vi "Untitled 1.vi"(11 "ZXing Options in":refnum<class "ZXing Options.lvclass">) -> (3 "ZXing Options out":refnum<class "ZXing Options.lvclass">)   [LabVIEW 2020, in "feature_detection.lvlib" / "ZXing Options.lvclass"]
uses:
  ZXing Options.lvclass
  ZXing Options.lvclass/ZXing Options.ctl
panel:
  in  "Ring":u8(ring) items=["ASCII", "ISO8859_1", "ISO8859_2", "ISO8859_3", "ISO8859_4", "ISO8859_5", "ISO8859_6", "ISO8859_7", "ISO8859_8", "ISO8859_9", "ISO8859_10", "ISO8859_11", "ISO8859_13", "ISO8859_14", "ISO8859_15", "ISO8859_16", "Cp437", "Cp1250", "Cp1251", "Cp1252", "Cp1256", "Shift_JIS", "Big5", "GB2312", "GB18030", "EUC_JP", "EUC_KR", "UTF16BE", "UTF8", "UTF16LE", "UTF32BE", "UTF32LE", "BINARY"]
  out "string array":string[](array[string])
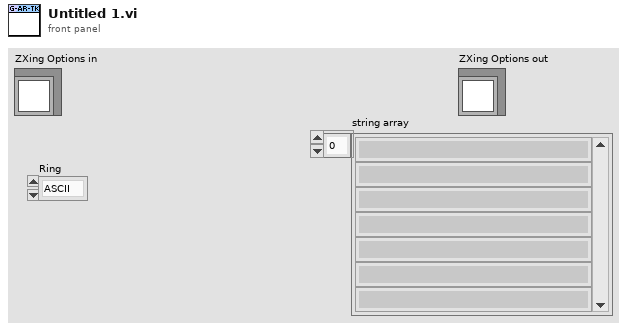
[diagram p1: front panel]
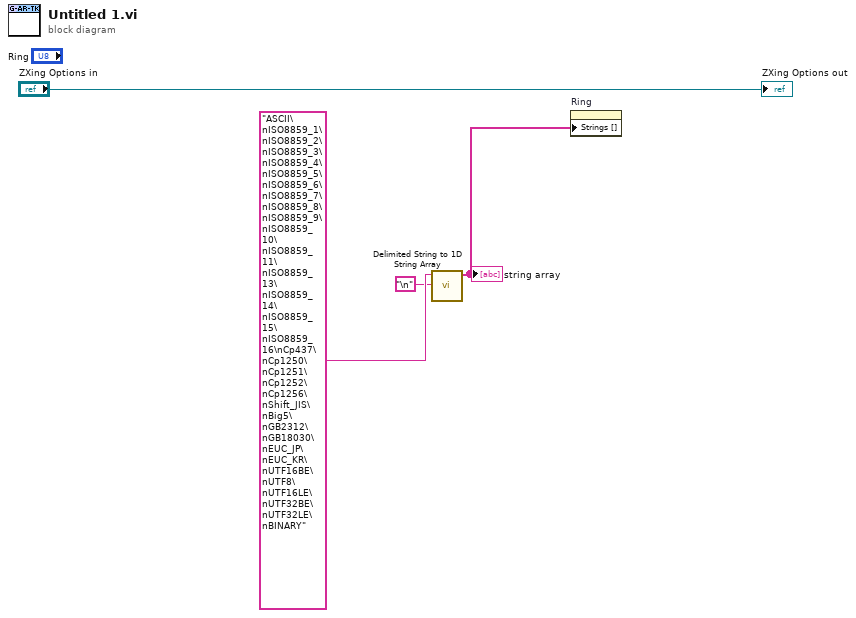
[diagram p0: block diagram]
diagram:
  n1 = call <vilib>:"Delimited String to 1D String Array.vi"("delimiter"="\n", "delimited string"="ASCII\nISO8859_1\nISO8859_2\nISO8859_3\nISO8859_4\nISO8859_5\nISO8859_6\nISO8859_7\nISO8859_8\nISO8859_9\nISO8859_10\nISO8859_11\nISO8859_13\nISO8859_14\nISO8859_15\nISO8859_16\nCp437\nCp1250\nCp1251\nCp1252\nCp1256\nShift_JIS\nBig5\nGB2312\nGB18030\nEUC_JP\nEUC_KR\nUTF16BE\nUTF8\nUTF16LE\nUTF32BE\nUTF32LE\nBINARY") -> ("string array"=w1:string[])  [unwired: 9 in]
  "string array" <- w1
  n2 = property on="Ring" class="Ring (strict)"("Strings []"=w1) -> ()  [unwired: 2 in, 2 out]
  "ZXing Options out" <- "ZXing Options in"
